vi "Translate Tip.vi"(8 "error in (no error)":errorcluster, 10 "Coordinate":cluster{"X":dbl, "Y":dbl}, 11 "SceneObject in":refnum<vi>) -> (0 "error out":errorcluster)   [LabVIEW 2016]
doc: "This VI moves the 3D tip to the specified coordinate."
uses:
  Global Variables.vi
  <vilib>/picture/3D Picture Control/NI_3D Picture Control.lvlib
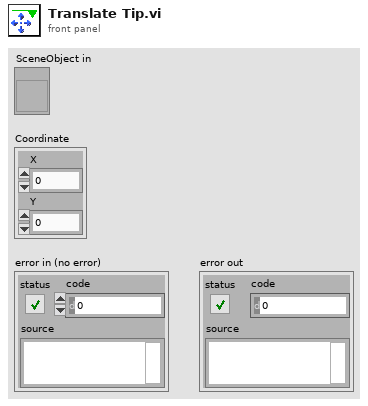
[diagram p1: front panel]
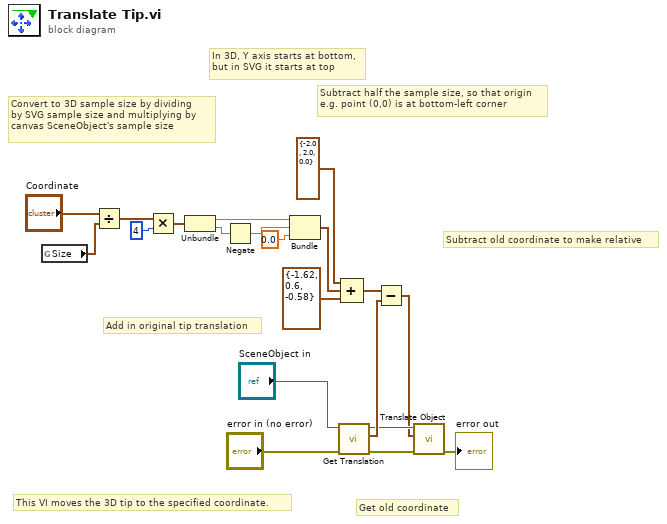
[diagram p0: block diagram]
diagram:
  # "Get old coordinate"
  # "Subtract old coordinate to make relative"
  # "Add in original tip translation"
  # "Subtract half the sample size, so that origin\ne.g. point (0,0) is at bottom-left corner"
  # "In 3D, Y axis starts at bottom,\nbut in SVG it starts at top"
  # "Convert to 3D sample size by dividing\nby SVG sample size and multiplying by\ncanvas SceneObject's sample size"
  # "This VI moves the 3D tip to the specified coordinate."
  n1 = global read "Global Variables.vi" "Size"() -> (w8:cluster{"Width":dbl, "Height":dbl})
  n2 = Divide(x="Coordinate", y=w8) -> (x/y=w11:cluster{dbl, dbl})
  n3 = Multiply(x=w11, y=4 ("Y")) -> (x*y=w13:cluster{dbl, dbl})
  n4 = Unbundle(w13) -> (w10:dbl, w15:dbl)
  n5 = Negate(x=w15) -> (-x=w16:dbl)
  n6 = Bundle(w10, w16, "Y"=0.0) -> (w17:cluster{dbl, dbl, "Y":dbl})  [unwired: 1 in]
  n7 = call <vilib>:"Get Translation.vi"("error in (no error)"="error in (no error)", "Scene Object"="SceneObject in") -> ("error out"=w6:errorcluster, "Transformation:Get Translation"=w14:cluster{"X":sgl, "Y":sgl, "Z":sgl}, "Scene Object"=w7:refnum<vi>)  [unwired: 7 in]
  n8 = Compound Arithmetic op=ADD(cluster{"X":dbl, "Y":dbl, "Z":dbl} {"X"=-2.0, "Y"=2.0, "Z"=0.0} ("Initial Coordinate"), w17, cluster{"X":dbl, "Y":dbl, "Z":dbl} {"X"=-1.62, "Y"=0.6, "Z"=-0.58} ("Initial Coordinate")) -> (w19:cluster{dbl, dbl, dbl})
  n9 = Subtract(x=w19, y=w14) -> (x-y=w4:cluster{dbl, dbl, dbl})
  n10 = call <vilib>:"Translate Object.vi"("error in (no error)"=w6, "Translation"=w4, "Scene.Object In"=w7) -> ("error out"=→"error out":errorcluster)  [unwired: 7 in, 1 out]
